vi "Update_SourceItem_from_Linker.vi"(8 "error in (no error)":errorcluster, 10 "linkerInfo":T2, 11 "AB_Source_Library in":refnum<class "AB_Source_Library.lvclass">) -> (0 "error out":errorcluster, 3 "AB_Source_Library out":refnum<class "AB_Source_Library.lvclass">)   [LabVIEW 2020, in "AB_Source_Library.lvclass"]
uses:
  <vilib>/AppBuilder/AB_Classes/Source/Library/AB_Source_Library.lvclass
  e:/builds/penguin/labview/branches/2020/dev/dist/vi.lib/AppBuilder/AB_Classes/Source/AB_Source.lvclass
  <vilib>/Utility/lvfile.llb/LVFileType.ctl
  <vilib>/AppBuilder/AB_Classes/Source/AB_Source.lvclass
  <vilib>/Utility/lvfile.llb/NI_FileType.lvlib
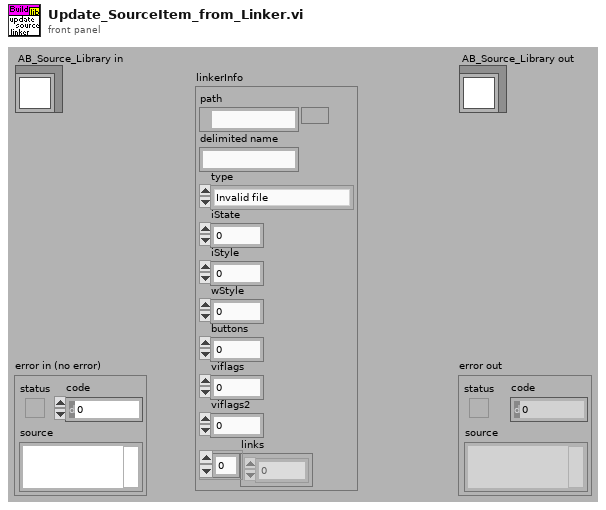
[diagram p1: front panel]
types:
  T1 = typedef "NI_FileType.lvlib/LVFileType.ctl" = enum32{"Invalid file", "Unknown type", "Instrument", "Control", "Polymorphic VI", "Project", "Library", "LVClass", "XControl", "XNode", "Shared library", ".NET assembly", "ActiveX interface", "CIN", "Run-time menu", "Palette menu", "Help file", "LLB", "XNode Edit Dependency", "Class Private Data Control", "Statechart", "MathScript .m file", "Ladder Diagram", "LVLibp", "XNode Build Dependency"}
  T2 = cluster{"path":path, "delimited name":string, "type":T1, "iState":u32, "iStyle":u16, "wStyle":u16, "buttons":u16, "viflags":u32, "viflags2":u32, "links":u32[]}
  T3 = typedef "AB_Source.ctl" = cluster{"path":path, "itemID":string, "parentIndex":i32, "sourceInclusion":T4, "destinationIndex":i32, "properties":T5[], "newName":string, "lvfile":bool, "valid":bool, "eng_inBuild":bool, "eng_isNonVILink":bool, "Amalgamation":bool, "Amalgamation Piece":bool, "eng_delimitedName":string, "preventRename":bool}
  T4 = typedef "AB_Source_Inclusion.ctl" = enum16{"IncludeIfReferenced", "Include", "Exclude", "TopLevel"}
  T5 = typedef "AB_Source_Properties.ctl" = cluster{"sourcePropertyType":T6, "value":variant}
  T6 = typedef "AB_Source_Property_Type.ctl" = enum16{"Remove block diagram", "Remove front panel", "Password", "Window has title bar", "Show menu bar", "Show vertical scroll bar", "Show horizontal scroll bar", "Show toolbar", "Show Abort button", "Show fp when called", "Window behavior", "Allow user to close window", "Window run-time position", "Run when opened", "Allow debugging", "Auto error handling", "Generate guard code", "Use stack variables", "Expression folding", "Integer only", "Inline subVI"}
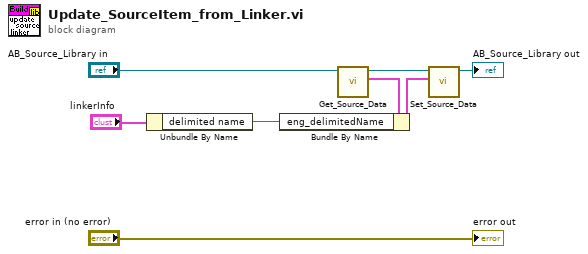
[diagram p0: block diagram]
diagram:
  n1 = Unbundle By Name("linkerInfo") -> ("delimited name"=w7:string)
  n2 = call <vilib>:"Get_Source_Data.vi"("Class in"="AB_Source_Library in") -> ("data"=w2:T3, "Class out"=w4:refnum<class "AB_Source_Library.lvclass">)  [unwired: 8 in, 1 out]
  n3 = Bundle By Name(cluster=w2, "eng_delimitedName"=w7) -> (w1:T3)
  n4 = call <vilib>:"Set_Source_Data.vi"("data"=w1, "Class in"=w4) -> ("Class out"=→"AB_Source_Library out":refnum<class "AB_Source_Library.lvclass">)  [unwired: 8 in, 1 out]
  "error out" <- "error in (no error)"
